vi "sv_Buffer Specified Cycles.vi"(0 "inital buffered x[n]":dbl[](array[numeric]), 1 "reset? (True)":bool=TRUE, 5 "x[n]":dbl[](array[numeric]) format="%.2f", 7 "fs":i32=1, 9 "integration cycles":u32) -> (4 "buffered x[n] for analysis":dbl[](array[numeric]), 6 "buffered x[n]":dbl[](array[numeric]))   [LabVIEW 2017]
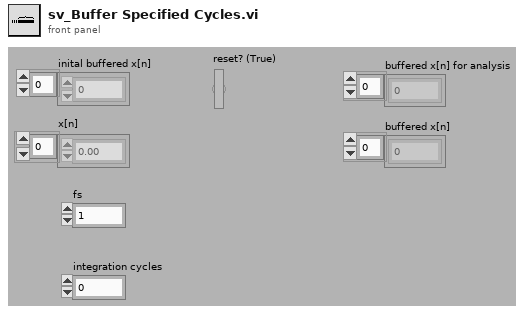
[diagram p1: front panel]
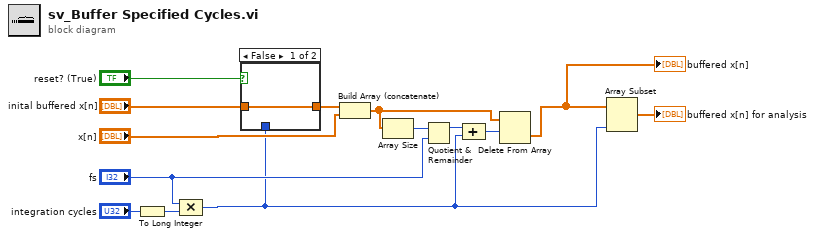
[diagram p0: block diagram]
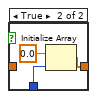
[diagram p2: hidden frame]
diagram:
  n1 = To Long Integer(number="integration cycles") -> (32bit integer=w11:i32)
  n2 = Compound Arithmetic op=MULTIPLY("fs", w11) -> (w10:i32)
  n3 = case shown="False" "reset? (True)" {
    tunnel: [w15 w17] -> w3
    tunnel: "inital buffered x[n]" -> [w15 _]
    tunnel: w10 -> [_ w16]
    frame False {
    }
    frame True {
      n4 = Initialize Array(0.0 ("element"), w16) -> (w17:dbl[])
    }
  }
  n5 = Build Array (concatenate)(w3, "x[n]") -> (w2:dbl[])
  n6 = Array Size(array=w2) -> (size(s)=w6:i32)
  n7 = Quotient & Remainder(x=w6, y="fs") -> (x-y*floor(x/y)=w5:i32)  [unwired: 1 out]
  n8 = Compound Arithmetic op=ADD(w5, w10) -> (w4:i32)
  n9 = Delete From Array(array=w2, length=w4) -> (deleted portion=w1:dbl[])  [unwired: 1 in, 1 out]
  "buffered x[n]" <- w1
  n10 = Array Subset(array=w1, length=w10) -> (→"buffered x[n] for analysis":dbl[])  [unwired: 1 in]
